vi "ArcadeArmControl.vi"(8 "error in (no error)":errorcluster, 9 "Speed Multipliers":cluster{"X":dbl, "Y":dbl, "Wrist":dbl}, 10 "X/Y Stick":cluster{"X":dbl, "Y":dbl}, 11 "Wrist Stick":cluster{"X":dbl, "Y":dbl}) -> (0 "error out":errorcluster)   [LabVIEW 2014]
uses:
  Robot Global Data.vi
panel:
  in  "Claw Operation":enum16{"Open", "Close", "Continue", "Stop"}(ring)
  in  "Claw %VBus":dbl=0.7
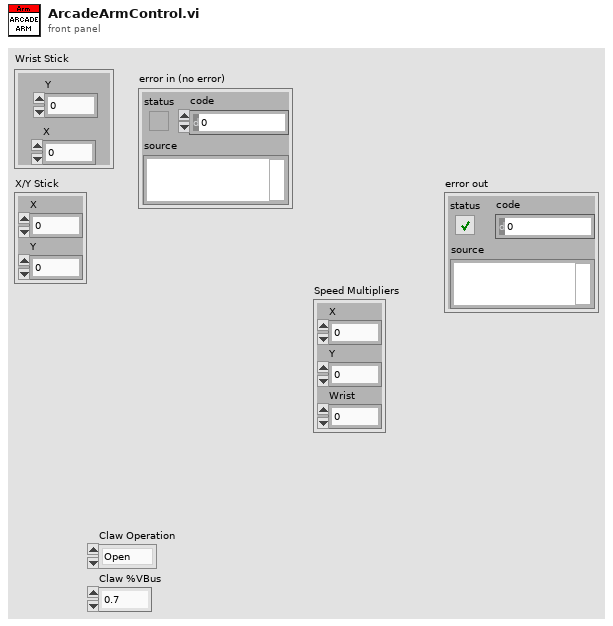
[diagram p1: front panel]
types:
  T1 = typedef "WPI_MotorControlDeviceRef.ctl" = cluster{"DeviceStatus":errorcluster, "Type":T2, "PWM":cluster{"Controller":T3, "PWM Channel":T4, "DeadBand":T5}, "CAN":cluster{"Device Number":u8, "Control Mode":T6, "Semaphore":T7, "Max Vout":dbl, "TalonSRX Control Mode":T8}, "Invert":bool, "TransformRef":T9, "InvTransformRef":T9}
  T2 = typedef "WPI_MotorControlType.ctl" = enum16{"PWM", "CAN", "CANTalonSRX"}
  T3 = typedef "FPGA_TypedefDigitalModule.ctl" = enum16{"Controller 1"}
  T4 = typedef "FPGA_DIOPWMChannel.ctl" = enum8{"PWM 0", "PWM 1", "PWM 2", "PWM 3", "PWM 4", "PWM 5", "PWM 6", "PWM 7", "PWM 8", "PWM 9", "PWM MXP 0", "PWM MXP 1", "PWM MXP 2", "PWM MXP 3", "PWM MXP 4", "PWM MXP 5", "PWM MXP 6", "PWM MXP 7", "PWM MXP 8", "PWM MXP 9", "Invalid"}
  T5 = typedef "WPI_PWMDeadband.ctl" = cluster{"Name":string, "maxPositivePwm":i32, "minPositivePwm":i32, "centerPwm":i32, "maxNegativePwm":i32, "minNegativePwm":i32, "angularRange":u16}
  T6 = typedef "WPI_CANJaguar_ControlMode.ctl" = enum8{"Percent VBus", "Current", "Speed", "Position", "Voltage"}
  T7 = typedef "Semaphore RefNum" = refnum<k1>
  T8 = typedef "WPI_CANTalonSRX_APIControlMode.ctl" = enum8{"Percent VBus", "Speed", "Position", "Slave", "Unchanged / Invalid"}
  T9 = typedef "WPI_PWMTransform_ConPane.ctl" = refnum<vi>
  T10 = typedef "WPI_CANTalonSRX_GlobalStatus.ctl" = cluster{"Applied Throttle":dbl, "Module Enabled":bool, "CAN Error":errorcluster, "Closed Loop Error":dbl, "Forward Limit Switch Closed":bool, "Reverse Limit Switch Closed":bool, "Sensor Position":dbl, "Sensor Velocity":dbl, "Current":dbl, "Sticky Fault - Over Temp":bool, "Sticky Fault - Under Voltage":bool, "Sticky Fault - Forward Limit":bool, "Sticky Fault - Reverse Limit":bool, "Sticky Fault - Forward Soft Limit":bool, "Sticky Fault - Reverse Soft Limit":bool, "Brake is Enabled":bool, "Encoder Position":dbl, "Encoder Velocity":dbl, "Encoder Index Count":dbl, "Encoder A Pin State":bool, "Encoder B Pin State":bool, "Encoder Index Pin State":bool, "Analog In":dbl, "Analog In Velocity":dbl, "Temperature (C)":dbl, "Battery Voltage":dbl}
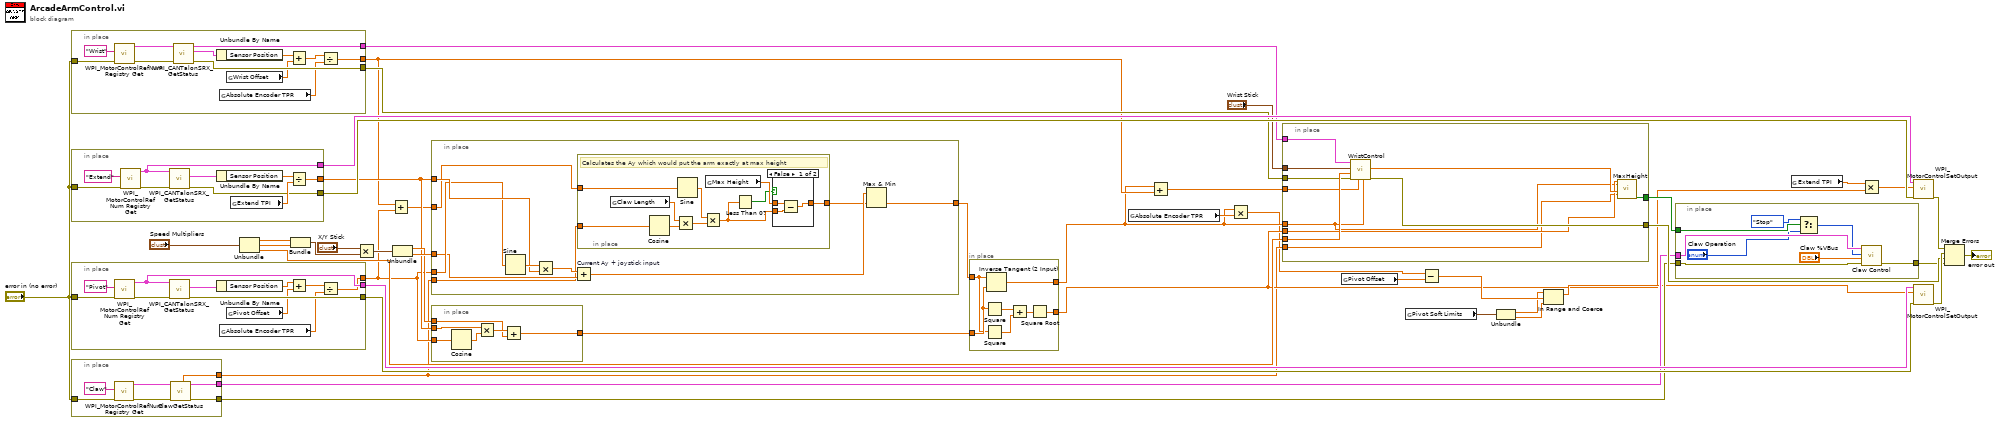
[diagram p0: block diagram]
diagram:
  n1 = in-place {
    in-place-border: "error in (no error)" -> [w56]
    in-place-border: [w54] -> w17
    in-place-border: [w52] -> w7
    in-place-border: [w49] -> w18
    n2 = call <vilib>:"WPI_MotorControlRefNum Registry Get.vi"("error in (no error)"=w56, "refnum name"="Wrist") -> ("error out"=w55:errorcluster, "MotorControlDevRef"=w53:T1)  [unwired: 8 in]
    n3 = call <vilib>:"WPI_CANTalonSRX_GetStatus.vi"("error in (no error)"=w55, "CAN Talon SRX Ref"=w53) -> ("error out"=w54:errorcluster, "Talon SRX Status"=w57:T10, "CAN Talon SRX Ref Out"=w49:T1)  [unwired: 7 in]
    n4 = Unbundle By Name(w57) -> ("Sensor Position"=w47:dbl)
    n5 = global read "Robot Global Data.vi" "Absolute Encoder TPR"() -> (w50:dbl)
    n6 = global read "Robot Global Data.vi" "Wrist Offset"() -> (w48:dbl)
    n7 = Add(x=w47, y=w48) -> (x+y=w46:dbl)
    n8 = Divide(x=w46, y=w50) -> (x/y=w52:dbl)
  }
  n9 = in-place {
    in-place-border: "error in (no error)" -> [w66]
    in-place-border: [w61] -> w10
    in-place-border: [w59] -> w38
    in-place-border: [w58] -> w39
    n10 = call <vilib>:"WPI_MotorControlRefNum Registry Get.vi"("error in (no error)"=w66, "refnum name"="Extend") -> ("error out"=w63:errorcluster, "MotorControlDevRef"=w59:T1)  [unwired: 8 in]
    n11 = call <vilib>:"WPI_CANTalonSRX_GetStatus.vi"("error in (no error)"=w63, "CAN Talon SRX Ref"=w59) -> ("error out"=w58:errorcluster, "Talon SRX Status"=w64:T10)  [unwired: 7 in, 1 out]
    n12 = Unbundle By Name(w64) -> ("Sensor Position"=w62:dbl)
    n13 = global read "Robot Global Data.vi" "Extend TPI"() -> (w60:dbl)
    n14 = Divide(x=w62, y=w60) -> (x/y=w61:dbl)
  }
  n15 = in-place {
    in-place-border: "error in (no error)" -> [w77]
    in-place-border: [w75] -> w40
    in-place-border: [w74] -> w41
    in-place-border: [w71] -> w9
    n16 = call <vilib>:"WPI_MotorControlRefNum Registry Get.vi"("error in (no error)"=w77, "refnum name"="Pivot") -> ("error out"=w76:errorcluster, "MotorControlDevRef"=w75:T1)  [unwired: 8 in]
    n17 = call <vilib>:"WPI_CANTalonSRX_GetStatus.vi"("error in (no error)"=w76, "CAN Talon SRX Ref"=w75) -> ("error out"=w74:errorcluster, "Talon SRX Status"=w73:T10)  [unwired: 7 in, 1 out]
    n18 = Unbundle By Name(w73) -> ("Sensor Position"=w69:dbl)
    n19 = global read "Robot Global Data.vi" "Absolute Encoder TPR"() -> (w72:dbl)
    n20 = global read "Robot Global Data.vi" "Pivot Offset"() -> (w68:dbl)
    n21 = Add(x=w69, y=w68) -> (x+y=w67:dbl)
    n22 = Divide(x=w67, y=w72) -> (x/y=w71:dbl)
  }
  n23 = in-place {
    in-place-border: [w84] -> w3
    in-place-border: "error in (no error)" -> [w80]
    in-place-border: [w79] -> w12
    in-place-border: [w78] -> w14
    n24 = call <vilib>:"WPI_MotorControlRefNum Registry Get.vi"("error in (no error)"=w80, "refnum name"="Claw") -> ("error out"=w81:errorcluster, "MotorControlDevRef"=w82:T1)  [unwired: 8 in]
    n25 = call "ClawGetStatus.vi"("error in (no error)"=w81, "MotorControlDevRef"=w82) -> ("error out"=w79:errorcluster, "MotorControlDevRef"=w78:T1, "Claw Angle"=w84:dbl)  [unwired: 5 in, 2 out]
  }
  n26 = Unbundle("Speed Multipliers") -> ("X"=w28:dbl, "Y"=w27:dbl, "Wrist"=w19:dbl)
  n27 = Bundle("X"=w28, "Y"=w27) -> (w26:cluster{"X":dbl, "Y":dbl})  [unwired: 1 in]
  n28 = Multiply(x="X/Y Stick", y=w26) -> (x*y=w43:cluster{"X":dbl, "Y":dbl})
  n29 = Add(x=w7, y=w9) -> (x+y=w8:dbl)
  n30 = Unbundle(w43) -> ("X"=w42:dbl, "Y"=w44:dbl)
  n31 = in-place {
    in-place-border: w10 -> [w93]
    in-place-border: w8 -> [w88]
    in-place-border: w9 -> [w92]
    in-place-border: w44 -> [w91]
    in-place-border: [w86] -> w33
    in-place-border: w3 -> [w87]
    n32 = Sine(x=w92) -> (sin(x)=w94:dbl)
    n33 = Multiply(x=w94, y=w93) -> (x*y=w89:dbl)
    n34 = Add "Current Ay + joystick input"(x=w89, y=w91) -> (x+y=w90:dbl)
    n35 = in-place {
      in-place-border: w88 -> [w97]
      in-place-border: w87 -> [w96]
      in-place-border: [w95] -> w85
      # "Calculates the Ay which would put the arm exactly at max height"
      n36 = global read "Robot Global Data.vi" "Claw Length"() -> (w102:dbl)
      n37 = Cosine(x=w96) -> (cos(x)=w100:dbl)
      n38 = Multiply(x=w102, y=w100) -> (x*y=w101:dbl)
      n39 = Sine(x=w97) -> (sin(x)=w104:dbl)
      n40 = Multiply(x=w104, y=w101) -> (x*y=w99:dbl)
      n41 = global read "Robot Global Data.vi" "Max Height"() -> (w103:dbl)
      n42 = Less Than 0?(x=w99) -> (x < 0?=w98:bool)
      n43 = case shown="False" w98 {
        tunnel: w103 -> [w107 w108]
        tunnel: w99 -> [w106 _]
        tunnel: [w105 w108] -> w95
        frame False {
          n44 = Subtract(x=w107, y=w106) -> (x-y=w105:dbl)
        }
        frame True {
        }
      }
    }
    n45 = Max & Min(x=w90, y=w85) -> (min(x,y)=w86:dbl)  [unwired: 1 out]
  }
  n46 = in-place {
    in-place-border: w9 -> [w114]
    in-place-border: w10 -> [w112]
    in-place-border: w42 -> [w110]
    in-place-border: [w109] -> w34
    n47 = Cosine(x=w114) -> (cos(x)=w113:dbl)
    n48 = Multiply(x=w112, y=w113) -> (x*y=w111:dbl)
    n49 = Add(x=w111, y=w110) -> (x+y=w109:dbl)
  }
  n50 = in-place {
    in-place-border: [w121] -> w2
    in-place-border: w34 -> [w120]
    in-place-border: w33 -> [w119]
    in-place-border: [w115] -> w4
    n51 = Square(x=w120) -> (x^2=w117:dbl)
    n52 = Square(x=w119) -> (x^2=w118:dbl)
    n53 = Inverse Tangent (2 Input)(1:w120, 2:w119) -> (0:w121:dbl)
    n54 = Add(x=w117, y=w118) -> (x+y=w116:dbl)
    n55 = Square Root(x=w116) -> (sqrt(x)=w115:dbl)
  }
  n56 = global read "Robot Global Data.vi" "Absolute Encoder TPR"() -> (w30:dbl)
  n57 = Add(x=w2, y=w7) -> (x+y=w6:dbl)
  n58 = Multiply(x=w2, y=w30) -> (x*y=w1:dbl)
  n59 = in-place {
    in-place-border: "Wrist Stick" -> [w132]
    in-place-border: w19 -> [w131]
    in-place-border: w18 -> [w130]
    in-place-border: w17 -> [w129]
    in-place-border: [w128] -> w16
    in-place-border: [w127] -> w11
    in-place-border: w6 -> [w126]
    in-place-border: w4 -> [w124]
    in-place-border: w3 -> [w123]
    in-place-border: w2 -> [w122]
    n60 = call "WristControl.vi"("Pivot Angle"=w122, "Wrist Angle (relative to ground)"=w126, "error in (no error)"=w129, "Wrist Multiplier"=w131, "Wrist Stick"=w132, "MotorControlDevRef"=w130) -> ("error out"=w128:errorcluster, "Target Wrist Angle (relative to ground)"=w125:dbl)  [unwired: 3 in, 1 out]
    n61 = call "MaxHeight.vi"("Extension Length"=w124, "Pivot Angle"=w122, "Wrist Angle (relative to ground)"=w125, "Claw Angle"=w123) -> ("Disable Claw Close"=w127:bool)  [unwired: 10 in, 5 out]
  }
  n62 = global read "Robot Global Data.vi" "Pivot Offset"() -> (w25:dbl)
  n63 = global read "Robot Global Data.vi" "Pivot Soft Limits"() -> (w23:cluster{"Forward":dbl, "Reverse":dbl})
  n64 = Subtract(x=w1, y=w25) -> (x-y=w24:dbl)
  n65 = Unbundle(w23) -> ("Forward"=w22:dbl, "Reverse"=w21:dbl)
  n66 = In Range and Coerce(upper limit=w22, x=w24, lower limit=w21) -> (coerced(x)=w5:dbl)  [unwired: 1 out]
  n67 = in-place {
    in-place-border: w14 -> [w140]
    in-place-border: w11 -> [w138]
    in-place-border: w12 -> [w134]
    in-place-border: [w133] -> w13
    n68 = Select(t=enum16{"Open", "Close", "Continue", "Stop"}."Stop", s=w138, f="Claw Operation") -> (s? t:f=w135:enum16{"Open", "Close", "Continue", "Stop"})
    n69 = call "Claw Control.vi"("error in (no error)"=w134, "%VBus"="Claw %VBus", "Operation"=w135, "MotorControlDevRef"=w140) -> ("error out"=w133:errorcluster)  [unwired: 4 in, 1 out]
  }
  n70 = global read "Robot Global Data.vi" "Extend TPI"() -> (w31:dbl)
  n71 = Multiply(x=w31, y=w4) -> (x*y=w32:dbl)
  n72 = call <vilib>:"WPI_MotorControlSetOutput.vi"("error in (no error)"=w39, "Output"=w32, "MotorControlDevRef"=w38) -> ("error out"=w37:errorcluster)  [unwired: 6 in, 2 out]
  n73 = call <vilib>:"WPI_MotorControlSetOutput.vi"("error in (no error)"=w41, "Output"=w5, "MotorControlDevRef"=w40) -> ("error out"=w36:errorcluster)  [unwired: 6 in, 2 out]
  n74 = Merge Errors(w37, w36, w16, w13) -> (→"error out":errorcluster)
